vi "Get Custom Device Ref.vi"(9 "Custom Device GUID_Disabled":string, 10 "Custom Device GUID":string, 11 "Section Ptr":T1 format="%.0x") -> (0 "error out":errorcluster, 2 "Custom Device Ref":T1 format="%.0x", 3 "Section Ref out":T1 format="%.0x")   [LabVIEW 2025, in "Protection and Counter Addon System Explorer.lvlib"]
uses:
  Protection and Counter Addon System Explorer.lvlib
  <vilib>/NI VeriStand/Custom Device API/Custom Device Item Ref.ctl
  <vilib>/NI VeriStand/Custom Device Tools/Custom Device Utility Library/Search Direction.ctl
  <vilib>/NI VeriStand/Custom Device Tools/Custom Device Utility Library/NI VeriStand - Search for Item by GUID.vi
  <vilib>/NI VeriStand/Custom Device Tools/Custom Device Utility Library/Custom Device Utility Library.lvlib
  <vilib>/NI VeriStand/Custom Device API/Custom Device API.lvlib
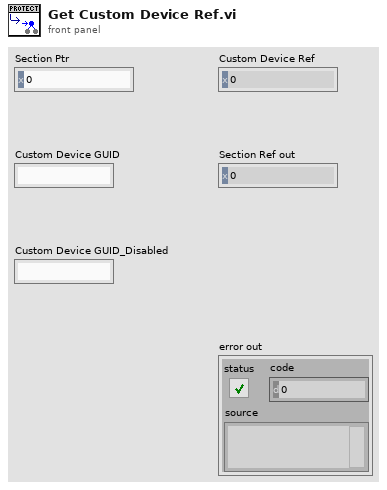
[diagram p1: front panel]
types:
  T1 = typedef "Custom Device API.lvlib/Custom Device Item Ref.ctl" = u64
  T2 = typedef "Custom Device Utility Library.lvlib/Search Direction.ctl" = enum16{"Down", "Up"}
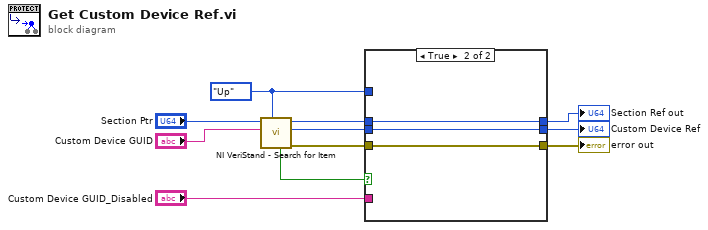
[diagram p0: block diagram]
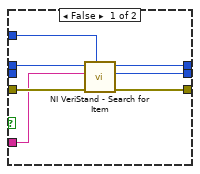
[diagram p2: hidden frame]
diagram:
  w1 = Search_Direction."Up" ("Direction (Down)")
  n1 = call-poly <vilib>:"NI VeriStand - Search for Item.vi"("Direction (Down)"=w1, "Item GUID"="Custom Device GUID", "Section Ref in"="Section Ptr") -> ("error out"=w2:errorcluster, "Item Ref"=w9:T1, "Section Ref out"=w3:T1, "Found"=w6:bool)  [unwired: 5 in]
  n2 = case shown="True" w6 {
    tunnel: w1 -> [w18 _]
    tunnel: w2 -> [w17 w21]
    tunnel: w3 -> [w16 w20]
    tunnel: [w15 w20] -> w5
    tunnel: "Custom Device GUID_Disabled" -> [w14 _]
    tunnel: [w13 w19] -> w10
    tunnel: [w12 w21] -> w11
    tunnel: w9 -> [_ w19]
    frame False {
      n3 = call-poly <vilib>:"NI VeriStand - Search for Item.vi"("Direction (Down)"=w18, "error in"=w17, "Item GUID"=w14, "Section Ref in"=w16) -> ("error out"=w12:errorcluster, "Item Ref"=w13:T1, "Section Ref out"=w15:T1)  [unwired: 4 in, 1 out]
    }
    frame True {
    }
  }
  "error out" <- w11
  "Custom Device Ref" <- w10
  "Section Ref out" <- w5
